vi "SGUI Set Control Captions By Label.vi"(6 "error in":errorcluster, 8 "labels (empty)":string, 9 "captions (empty)":string) -> (7 "error out":errorcluster, 11 "control references out":refnum<vi>[](array[refnum]))   [LabVIEW 2020, in "varilib.lvlib"]
doc: "This VI sets caption(s) of control(s) designated by label(s) name string. Multiple can be assigned at once by using multiline string for both 'labels' and 'captions' inputs. One line per control.\n\nThi VI ignores input errors (will execute anyway) however will generate error if any of the named controls is not found or writting to it fails (invalid type of control)."
uses:
  varilib.lvlib
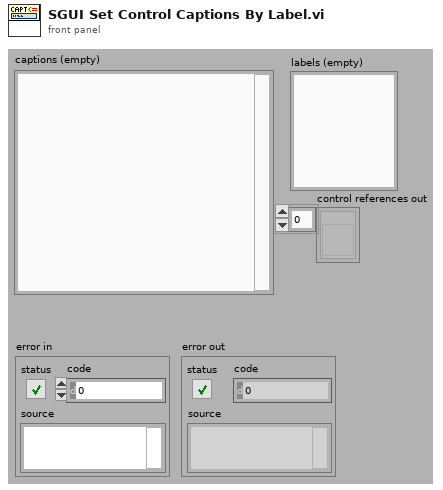
[diagram p1: front panel]
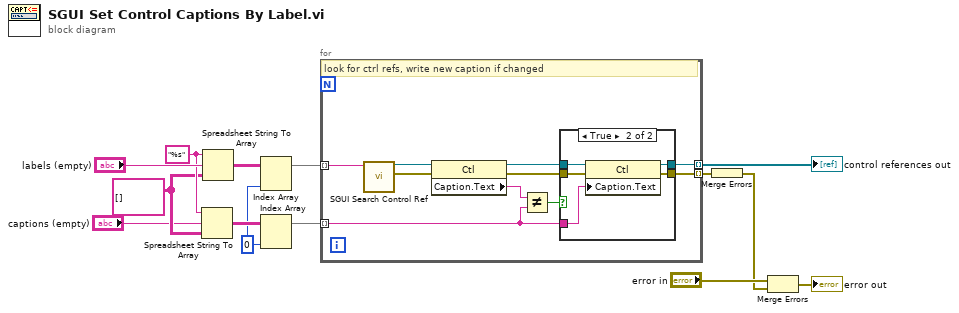
[diagram p0: block diagram]
diagram:
  w1 = 0 ("disabled index (col)")
  w6 = string[][] []
  w7 = "%s"
  n1 = Spreadsheet String To Array(format string=w7, spreadsheet string="captions (empty)", array type (2D Dbl)=w6) -> (array=w4:string[][])  [unwired: 1 in]
  n2 = Spreadsheet String To Array(format string=w7, spreadsheet string="labels (empty)", array type (2D Dbl)=w6) -> (array=w14:string[][])  [unwired: 1 in]
  n3 = Index Array(array=w14, index (col)=w1) -> (element=w3:string[])  [unwired: 1 in]
  n4 = Index Array(array=w4, index (col)=w1) -> (element=w2:string[])  [unwired: 1 in]
  n5 = for {
    tunnel: w3 -> [w24] mode=indexing
    tunnel: [w21] -> w12 mode=indexing
    tunnel: [w22] -> w13 mode=indexing
    tunnel: w2 -> [w17] mode=indexing
    # "look for ctrl refs, write new caption if changed"
    n6 = call "SGUI Search Control Ref.vi"("control label (empty)"=w24) -> ("error out"=w16:errorcluster, "control ref out"=w15:refnum<vi>)  [unwired: 8 in, 1 out]
    n7 = property class="Ctl"(reference=w15, error in=w16) -> (reference out=w20:refnum<vi>, error out=w23:errorcluster, "Caption.Text"=w18:string)
    n8 = Not Equal?(x=w18, y=w17) -> (x != y?=w19:bool)
    n9 = case shown="True" w19 {
      tunnel: w23 -> [w26 w31]
      tunnel: [w26 w30] -> w22
      tunnel: [w25 w29] -> w21
      tunnel: w20 -> [w25 w28]
      tunnel: w17 -> [_ w27]
      frame False {
      }
      frame True {
        n10 = property class="Ctl"(reference=w28, error in=w31, "Caption.Text"=w27) -> (reference out=w29:refnum<vi>, error out=w30:errorcluster)
      }
    }
  }
  "control references out" <- w12
  n11 = Merge Errors(w13) -> (w8:errorcluster)
  n12 = Merge Errors("error in", w8) -> (→"error out":errorcluster)
